vi "Clear Report Text.vi"(0 "report in":refnum<class "NI_Standard Report.lvclass">, 11 "error in (no error)":errorcluster) -> (4 "report out":refnum<class "NI_Standard Report.lvclass">, 15 "error out":errorcluster)   [LabVIEW 2017, in "NI_Standard Report.lvclass"]
doc: "Clears the text and related formatting information from the report. You cannot use this VI with Word and Excel reports."
uses:
  <vilib>/Utility/NIReport.llb/Standard Report/NI_Standard Report.lvclass
  <vilib>/Utility/NIReport.llb/Standard Report/NI_Standard Report.lvclass/NI_Standard Report.ctl
  <vilib>/Utility/NIReport.llb/NI_ReportGenerationCore.lvlib
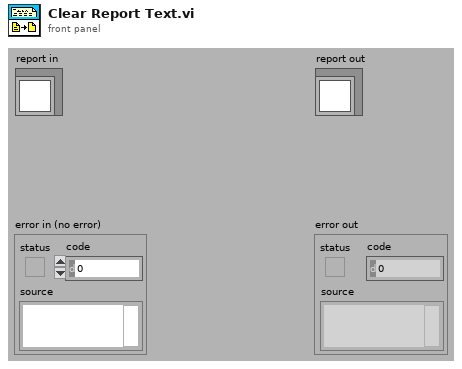
[diagram p1: front panel]
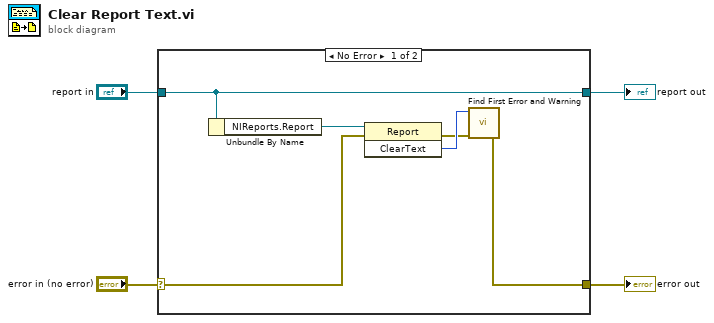
[diagram p0: block diagram]
diagram:
  n1 = case shown="No Error" "error in (no error)" {
    selector: "error in (no error)" -> [w6 w12]
    tunnel: [w5 w12] -> w3
    tunnel: [w7 w11] -> w1
    tunnel: "report in" -> [w7 w11]
    frame No Error {
      n2 = Unbundle By Name(w7) -> ("NIReports.Report"=w8:refnum<k7>)
      n3 = invoke class="Report" method="ClearText"(reference=w8, error in=w6) -> (error out=w9:errorcluster, "ClearText"=w10:i32)  [unwired: 1 in, 1 out]
      n4 = call <vilib>:"Find First Error and Warning.vi"("error in (no error)"=w9, "error code"=w10) -> ("error out"=w5:errorcluster)  [unwired: 1 in, 4 out]
    }
    frame Error {
    }
  }
  "error out" <- w3
  "report out" <- w1
